vi "PWM Test CB_TSFTS2.vi"(8 "error in (no error)":errorcluster, 10 "Message IN":string=" ") -> (0 "error out":errorcluster, 1 "Result (bool)":bool, 2 "Message OUT":string, 3 "ControlBoard OUT":refnum<visa-resource-name>)   [LabVIEW 2022 SP3]
uses:
  HMP4000 Communication/HMP4040_ChannelControl.ctl
  <vilib>/DAQmx/read.llb/DAQmx Read (Analog 1D Wfm NChan NSamp).vi
  <vilib>/DAQmx/miscellaneous.llb/DAQmx Fill In Error Info.vi
panel:
  out "Analysis Leg":i32
  out "Waveforms":T1
  out "Active Leg":i32
  out "Result (color)":u32(colorbox)
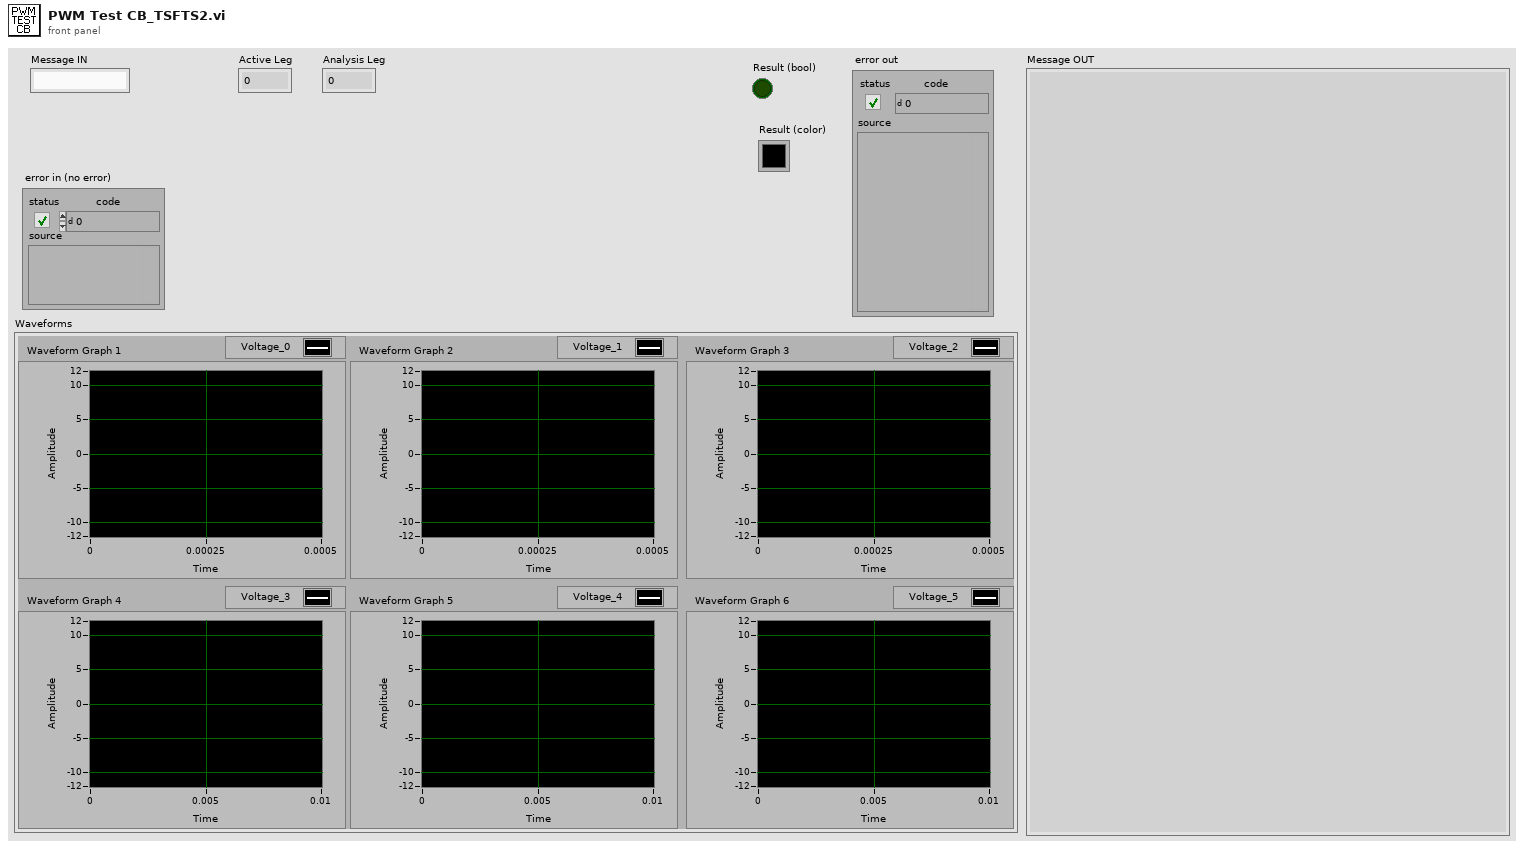
[diagram p1: front panel]
types:
  T1 = cluster{"Waveform Graph 1":waveform(dbl), "Waveform Graph 2":waveform(dbl), "Waveform Graph 3":waveform(dbl), "Waveform Graph 4":waveform(dbl), "Waveform Graph 5":waveform(dbl), "Waveform Graph 6":waveform(dbl)}
  T2 = typedef "HMP4040_ChannelControl.ctl" = cluster{"CH1 Voltage":dbl, "CH1 Current":dbl, "CH1 Output":bool, "CH2 Voltage":dbl, "CH2 Current":dbl, "CH2 Output":bool, "CH3 Voltage":dbl, "CH3 Current":dbl, "CH3 Output":bool, "CH4 Voltage":dbl, "CH4 Current":dbl, "CH4 Output":bool, "Master Output":bool}
  T3 = cluster{"data[0]":waveform(dbl), "data[1]":waveform(dbl), "data[2]":waveform(dbl), "data[3]":waveform(dbl), "data[4]":waveform(dbl), "data[5]":waveform(dbl)}
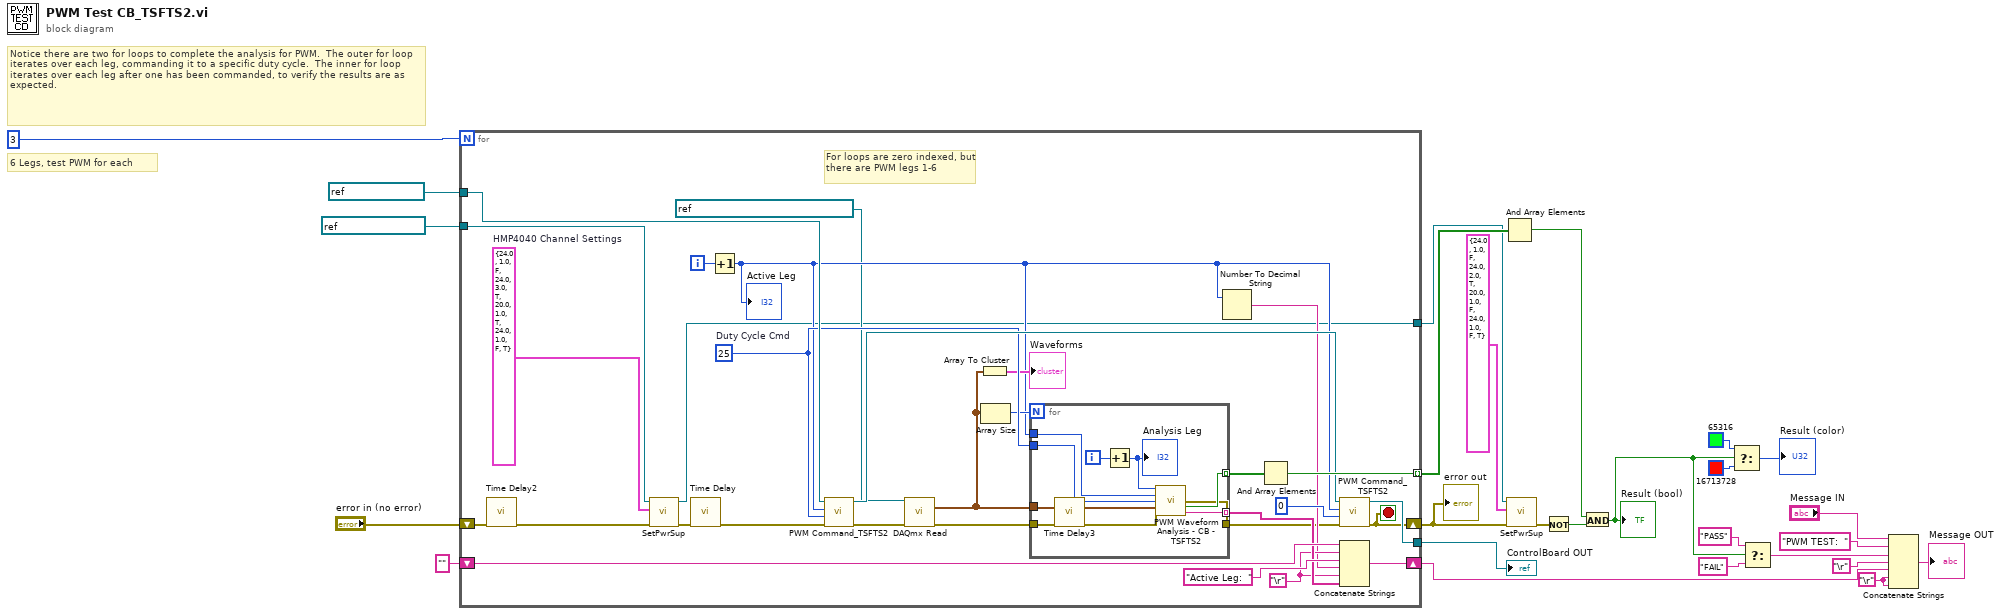
[diagram p0: block diagram]
diagram:
  w16 = "\r"
  # "Notice there are two for loops to complete the analysis for PWM.  The outer for loop iterates over each leg, commanding it to a specific duty cycle.  The inner for loop iterates over each leg after one has been commanded, to verify the results are as expected."
  # "6 Legs, test PWM for each"
  n1 = for {
    N: 3 -> [_]
    tunnel: refnum<visa-resource-name> "ControlBoard" ("ControlBoard_IN") -> [w51]
    tunnel: [w56] -> w26 mode=indexing
    shift-right: [w55] -> w14
    shift-left: "" -> [w54]
    tunnel: [w36] -> w4
    tunnel: refnum<visa-resource-name> "HMP4040_FTS2" ("HMP4040_IN") -> [w35]
    tunnel: [w44] -> w5
    shift-right: [w30] -> w2
    shift-left: "error in (no error)" -> [w28]
    i -> [w49]
    stop <- w30 stop-if-true
    w34 = T2 {"CH1 Voltage"=24.0, "CH1 Current"=1.0, "CH1 Output"=FALSE, "CH2 Voltage"=24.0, "CH2 Current"=3.0, "CH2 Output"=TRUE, "CH3 Voltage"=20.0, "CH3 Current"=1.0, "CH3 Output"=TRUE, "CH4 Voltage"=24.0, "CH4 Current"=1.0, "CH4 Output"=FALSE, "Master Output"=TRUE}  # HMP4040 Channel Settings
    w39 = "\r"
    w50 = 25  # Duty Cycle Cmd
    # "For loops are zero indexed, but there are PWM legs 1-6"
    n2 = call "Time Delay2"("error in (no error)"=w28) -> ("error out"=w27:errorcluster)  [unwired: 10 in]
    n3 = call "SetPwrSup.vi"("error in (no error)"=w27, "HMP4040 Channel Settings"=w34, "HMP4040 IN"=w35) -> ("error out"=w33:errorcluster, "HMP4040_OUT"=w36:refnum<visa-resource-name>)  [unwired: 7 in]
    n4 = call "Time Delay"("error in (no error)"=w33) -> ("error out"=w32:errorcluster)  [unwired: 10 in]
    n5 = Increment(x=w49) -> (x+1=w41:i32)
    "Active Leg" <- w41
    n6 = call "PWM Command_TSFTS2.vi"("error in (no error)"=w32, "Duty Cycle"=w50, "Leg"=w41, "VISA Refnum in"=w51) -> ("error out"=w43:errorcluster, "VISA Refnum out"=w52:refnum<visa-resource-name>)  [unwired: 5 in, 1 out]
    n7 = call-poly <vilib>:"DAQmx Read.vi"("task/channels in"=refnum<k21> "FTS2_PWMInput_CarrierBoard", "error in"=w43) -> ("data"=w45:waveform(dbl)[], "error out"=w31:errorcluster)  [unwired: 11 in, 1 out]
    n8 = Array To Cluster(array=w45) -> (cluster=→"Waveforms":T3)
    n9 = Array Size(array=w45) -> (size(s)=w46:i32)
    n10 = for {
      N: w46 -> [_]
      tunnel: w50 -> [w66]
      tunnel: w45 -> [w65]
      tunnel: w41 -> [w64]
      tunnel: [w61] -> w47 mode=indexing
      tunnel: [w60] -> w40 mode=indexing
      tunnel: w31 -> [w59]
      tunnel: [w57] -> w29
      i -> [w63]
      n11 = call "Time Delay3"("error in (no error)"=w59) -> ("error out"=w58:errorcluster)  [unwired: 10 in]
      n12 = Increment(x=w63) -> (x+1=w62:i32)
      "Analysis Leg" <- w62
      n13 = call "PWM Waveform Analysis - CB - TSFTS2.vi"("Analysis Leg"=w62, "Active Leg"=w64, "Duty Cycle"=w66, "Waveform"=w65, "error in (no error)"=w58) -> ("error out"=w57:errorcluster, "Result (Boolean)"=w61:bool, "Message"=w60:string)  [unwired: 8 in]
    }
    n14 = Number To Decimal String(number=w41) -> (decimal integer string=w38:string)  [unwired: 1 in]
    n15 = And Array Elements(Boolean array=w47) -> (logical AND=w56:bool)
    n16 = call "PWM Command_TSFTS2.vi"("error in (no error)"=w29, "Duty Cycle"=0, "Leg"=w41, "VISA Refnum in"=w52) -> ("error out"=w30:errorcluster, "VISA Refnum out"=w44:refnum<visa-resource-name>)  [unwired: 5 in, 1 out]
    n17 = Concatenate Strings(w54, w39, "Active Leg:  ", w38, w39, w40) -> (w55:string)
  }
  "error out" <- w2
  "ControlBoard OUT" <- w5
  n18 = And Array Elements(Boolean array=w26) -> (logical AND=w17:bool)
  n19 = call "SetPwrSup.vi"("error in (no error)"=w2, "HMP4040 Channel Settings"=T2 {"CH1 Voltage"=24.0, "CH1 Current"=1.0, "CH1 Output"=FALSE, "CH2 Voltage"=24.0, "CH2 Current"=2.0, "CH2 Output"=TRUE, "CH3 Voltage"=20.0, "CH3 Current"=1.0, "CH3 Output"=FALSE, "CH4 Voltage"=24.0, "CH4 Current"=1.0, "CH4 Output"=FALSE, "Master Output"=TRUE}, "HMP4040 IN"=w4) -> ("error out"=w1:errorcluster)  [unwired: 7 in, 1 out]
  n20 = Not(x=w1) -> (.not. x?=w19:bool)
  n21 = And(x=w17, y=w19) -> (x .and. y?=w18:bool)
  "Result (bool)" <- w18
  n22 = Select(t=u32 65316 ("Result (color)"), s=w18, f=u32 16713728 ("Result (color)")) -> (s? t:f=→"Result (color)":u32)
  n23 = Select(t="PASS", s=w18, f="FAIL") -> (s? t:f=w9:string)
  n24 = Concatenate Strings("Message IN", "PWM TEST:  ", w9, "\r", w14, w16, w16) -> (→"Message OUT":string)
